vi "create_image_array.vi"(7 "Border Size":i32=3, 8 "error in (no error)":errorcluster, 9 "Prefix":string, 10 "Image Type":T2 items=["Grayscale (U8)", "Grayscale (I16)", "Grayscale (SGL)", "Complex (CSG)", "RGB (U32)", "HSL (U32)", "RGB (U64)", "Grayscale (U16)"], 11 "Num Images":i32) -> (0 "error out":errorcluster, 3 "Image Array":T1[](array[typedef]))   [LabVIEW 2016]
doc: "Creates a vector of images. Images are named with the specified prefix + the image number."
uses:
  <vilib>/vision/Image Controls.llb/IMAQ Image.ctl
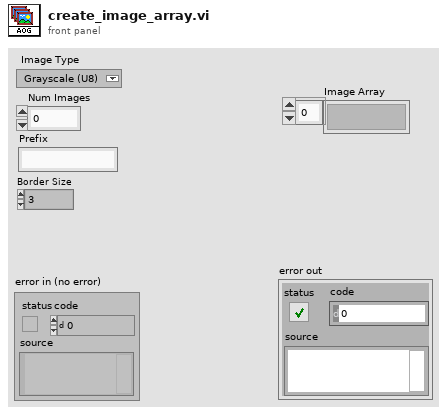
[diagram p1: front panel]
types:
  T1 = typedef "IMAQ Image.ctl" = refnum<image>
  T2 = typedef "Image Type" = u32
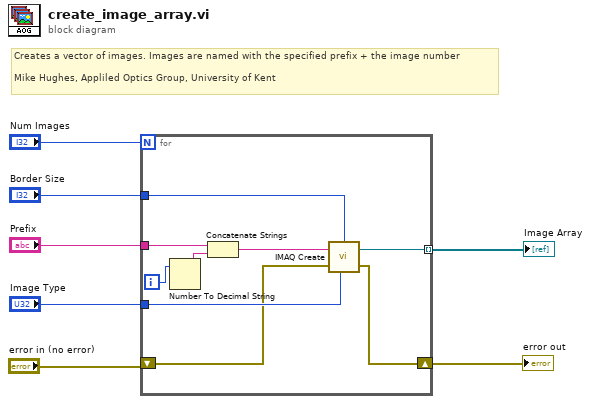
[diagram p0: block diagram]
diagram:
  # "Creates a vector of images. Images are named with the specified prefix + the image number\n\nMike Hughes, Appliled Optics Group, University of Kent"
  n1 = for {
    N: "Num Images" -> [_]
    tunnel: "Image Type" -> [w16]
    tunnel: "Prefix" -> [w15]
    tunnel: [w11] -> w3 mode=indexing
    tunnel: "Border Size" -> [w10]
    shift-right: [w8] -> w1
    shift-left: "error in (no error)" -> [w9]
    i -> [w13]
    n2 = Number To Decimal String(number=w13) -> (decimal integer string=w14:string)  [unwired: 1 in]
    n3 = Concatenate Strings(w15, w14) -> (w12:string)
    n4 = call "IMAQ Create"("Border Size"=w10, "Image Name"=w12, "Image Type"=w16, "error in (no error)"=w9) -> ("New Image"=w11:T1, "error out"=w8:errorcluster)  [unwired: 1 in]
  }
  "Image Array" <- w3
  "error out" <- w1
